vi "get_class_name.vi"(8 "error in (no error)":errorcluster, 11 "LabVIEW Object in":refnum<class>) -> (0 "error out":errorcluster, 3 "class name":string)   [LabVIEW 2014, in "LVCOOOP.lvlib" / "Lookup API.lvlib" / "Default Lookup.lvclass"]
uses:
  Default Lookup.lvclass
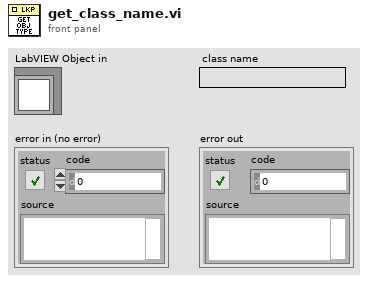
[diagram p1: front panel]
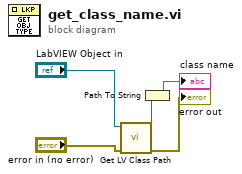
[diagram p0: block diagram]
diagram:
  n1 = call <vilib>:"Get LV Class Path.vi"("error in (no error)"="error in (no error)", "object"="LabVIEW Object in") -> ("error out"=→"error out":errorcluster, "class path"=w2:path)  [unwired: 8 in]
  n2 = Path To String(path=w2) -> (string=→"class name":string)
